vi "test_CCDSetAndGetTriggerIn.vi"(7 "Test should pass":bool=TRUE, 8 "error in":errorcluster, 9 "tear down connection":bool=TRUE, 10 "set-up a connection":bool=TRUE, 11 "device selection":enum16{"monochromator", "CCD", "SCD"}(ring)=enum."CCD") -> (0 "error out":errorcluster)   [LabVIEW 2023]
uses:
  Source/Classes/Mono/Monochromator.lvclass
  Source/Classes/CCD/CCD.lvclass
  Source/Classes/SCD/SCD.lvclass
  <vilib>/addons/_JKI Toolkits/Caraya/classes/Assert/Assert Equal Value and Type_Variant.vi
  <vilib>/addons/_JKI Toolkits/Caraya/classes/Assert/Assert Not Error.vi
  Source/Classes/GenericDevice/GenericDevice.lvclass
  <vilib>/addons/_JKI Toolkits/Caraya/classes/Test/Test.lvclass
  <vilib>/addons/_JKI Toolkits/Caraya/classes/Assert/Assert.lvclass
panel:
  # "Connector Pane"
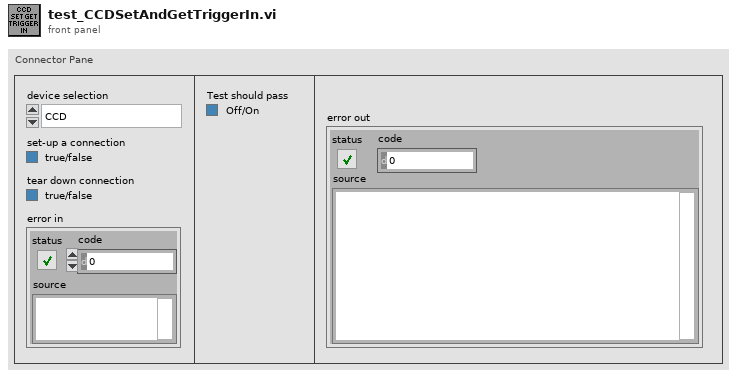
[diagram p1: front panel]
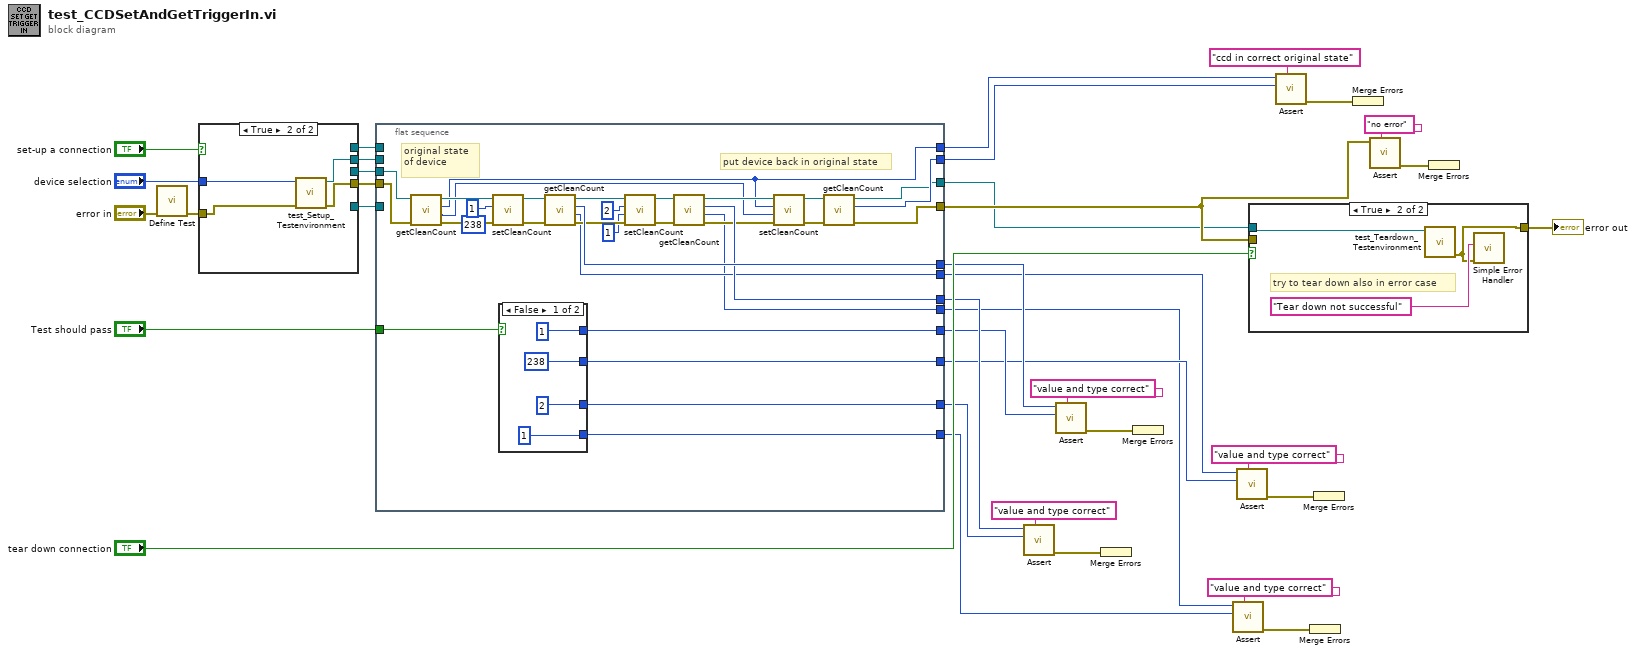
[diagram p0: block diagram]
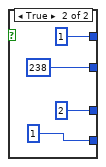
[diagram p2: hidden frame]
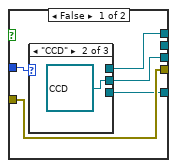
[diagram p3: hidden frame]
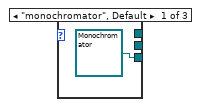
[diagram p4: hidden frame]
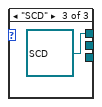
[diagram p5: hidden frame]
diagram:
  n1 = call <vilib>:"Define Test.vi"("error in (no error)"="error in") -> ("error out"=w28:errorcluster)  [unwired: 9 in, 1 out]
  n2 = case shown="True" "set-up a connection" {
    tunnel: w28 -> [w41 w48]
    tunnel: [w41 w47] -> w30
    tunnel: "device selection" -> [w40 w46]
    tunnel: [_ w45] -> w27
    tunnel: [w39 _] -> w26
    tunnel: [w38 _] -> w25
    tunnel: [w37 _] -> w24
    frame False {
      n3 = case shown="\"CCD\"" w40 {
        tunnel: [refnum<class "Monochromator.lvclass"> refnum ("Monochromator.lvclass") _ _] -> w39
        tunnel: [_ refnum<class "CCD.lvclass"> refnum ("CCD in") _] -> w38
        tunnel: [_ _ refnum<class "SCD.lvclass"> refnum ("SCD.lvclass")] -> w37
        frame "monochromator", Default {
        }
        frame "CCD" {
        }
        frame "SCD" {
        }
      }
    }
    frame True {
      n4 = call "test_Setup_Testenvironment.vi"("error in"=w48, "device selection"=w46) -> ("error out"=w47:errorcluster, "GenericDevice.lvclass"=w45:refnum<class "GenericDevice.lvclass">)  [unwired: 7 in, 1 out]
    }
  }
  n5 = flat-sequence {
    tunnel: w30 -> [w76]
    tunnel: w27 -> [_]
    tunnel: w26 -> [_]
    tunnel: w25 -> [w77]
    tunnel: w24 -> [_]
    tunnel: [w56] -> w19
    tunnel: "Test should pass" -> [w80]
    tunnel: [w57] -> w18
    tunnel: [w64] -> w17
    tunnel: [w79] -> w16
    tunnel: [w70] -> w15
    tunnel: [w78] -> w14
    tunnel: [w59] -> w11
    tunnel: [w58] -> w10
    tunnel: [w52] -> w6
    tunnel: [w51] -> w5
    tunnel: [w50] -> w2
    tunnel: [w49] -> w1
    frame #0 {
      # "put device back in original state"
      # "original state of device"
      n6 = call "getCleanCount.vi"("error in (no error)"=w76, "CCD in"=w77) -> ("error out"=w74:errorcluster, "mode"=w53:i32, "count"=w59:i32, "CCD out"=w75:refnum<class "CCD.lvclass">)  [unwired: 6 in]
      n7 = call "setCleanCount.vi"("error in (no error)"=w74, "mode"=238, "count"=1 ("exposure time [ms]"), "CCD in"=w75) -> ("error out"=w72:errorcluster, "CCD out"=w71:refnum<class "CCD.lvclass">)  [unwired: 4 in, 2 out]
      n8 = case shown="False" w80 {
        tunnel: [2 ("exposure time [ms]") 2 ("exposure time [ms]")] -> w79
        tunnel: [1 ("exposure time [ms]") 1 ("exposure time [ms]")] -> w78
        tunnel: [238 ("exposure time [ms]") 238 ("exposure time [ms]")] -> w52
        tunnel: [1 ("exposure time [ms]") 1 ("exposure time [ms]")] -> w49
        frame False {
        }
        frame True {
        }
      }
      n9 = call "getCleanCount.vi"("error in (no error)"=w72, "CCD in"=w71) -> ("error out"=w66:errorcluster, "mode"=w51:i32, "count"=w70:i32, "CCD out"=w67:refnum<class "CCD.lvclass">)  [unwired: 6 in]
      n10 = call "setCleanCount.vi"("error in (no error)"=w66, "mode"=1, "count"=2 ("exposure time [ms]"), "CCD in"=w67) -> ("error out"=w69:errorcluster, "CCD out"=w68:refnum<class "CCD.lvclass">)  [unwired: 4 in, 2 out]
      n11 = call "getCleanCount.vi"("error in (no error)"=w69, "CCD in"=w68) -> ("error out"=w61:errorcluster, "mode"=w50:i32, "count"=w64:i32, "CCD out"=w62:refnum<class "CCD.lvclass">)  [unwired: 6 in]
      n12 = call "setCleanCount.vi"("error in (no error)"=w61, "mode"=w53, "count"=w59, "CCD in"=w62) -> ("error out"=w63:errorcluster, "CCD out"=w60:refnum<class "CCD.lvclass">)  [unwired: 4 in, 2 out]
      n13 = call "getCleanCount.vi"("error in (no error)"=w63, "CCD in"=w60) -> ("error out"=w56:errorcluster, "count"=w58:i32, "CCD out"=w57:refnum<class "CCD.lvclass">)  [unwired: 6 in, 1 out]
    }
  }
  n14 = call-poly <vilib>:"Assert.vi"("Label"="value and type correct" ("Label (VI Title)"), "Y"=w16, "X"=w17) -> ("error out"=w34:errorcluster)  [unwired: 7 in, 1 out]
  n15 = call-poly <vilib>:"Assert.vi"("Label"="value and type correct" ("Label (VI Title)"), "Y"=w14, "X"=w15) -> ("error out"=w32:errorcluster)  [unwired: 7 in, 1 out]
  n16 = Merge Errors(w34) -> ()  [unwired: 1 out]
  n17 = Merge Errors(w32) -> ()  [unwired: 1 out]
  n18 = call-poly <vilib>:"Assert.vi"("Label"="value and type correct" ("Label (VI Title)"), "Y"=w1, "X"=w2) -> ("error out"=w4:errorcluster)  [unwired: 7 in, 1 out]
  n19 = call-poly <vilib>:"Assert.vi"("Label"="value and type correct" ("Label (VI Title)"), "Y"=w6, "X"=w5) -> ("error out"=w7:errorcluster)  [unwired: 7 in, 1 out]
  n20 = case shown="True" "tear down connection" {
    tunnel: w18 -> [_ w91]
    tunnel: [w89 w90] -> w9
    tunnel: w19 -> [w89 _]
    frame False {
    }
    frame True {
      # "try to tear down also in error case"
      n21 = call "test_Teardown_Testenvironment.vi"("GenericDevice.lvclass"=w91) -> ("error out"=w90:errorcluster)  [unwired: 9 in, 1 out]
      n22 = call <vilib>:"Simple Error Handler.vi"("error source (\" \")"="Tear down not successful" ("error source (\" \")"), "error in (no error)"=w90) -> ()  [unwired: 3 in, 5 out]
    }
  }
  "error out" <- w9
  n23 = call-poly <vilib>:"Assert.vi"("Label"="ccd in correct original state" ("Label (VI Title)"), "Y"=w10, "X"=w11) -> ("error out"=w13:errorcluster)  [unwired: 7 in, 1 out]
  n24 = Merge Errors(w4) -> ()  [unwired: 1 out]
  n25 = Merge Errors(w7) -> ()  [unwired: 1 out]
  n26 = Merge Errors(w13) -> ()  [unwired: 1 out]
  n27 = call-poly <vilib>:"Assert.vi"("Label"="no error" ("Label (VI Title)"), "Not Error?"=w19) -> ("error out"=w21:errorcluster)  [unwired: 8 in, 1 out]
  n28 = Merge Errors(w21) -> ()  [unwired: 1 out]
